vi "Analyzer.DVRtoRef.vi"(10 "Ref":T1) -> (2 "Ref":u32 format="%08x")   [LabVIEW 2022 SP3, in "Analyzer.lvclass"]
uses:
  Analyzer.lvclass
  Typedefs/PrivateData--Ref.ctl
  Typedefs/PrivateData--Cluster.ctl
  Typedefs/PublicEvents--Cluster.ctl
  Typedefs/Analyzer State--enum.ctl
  Typedefs/PublicEvents--Analyzer.NewEventMessage.ctl
  Typedefs/PrivateEvents--Cluster.ctl
  Typedefs/PrivateEvents--Analyzer.NewRequest.ctl
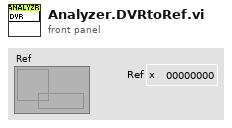
[diagram p1: front panel]
types:
  T1 = typedef "Analyzer.lvclass/PrivateData--Ref.ctl" = refnum<data-value>
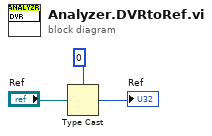
[diagram p0: block diagram]
diagram:
  n1 = Type Cast(type=u32 0 ("Ref"), x="Ref") -> (*(type *) &x=→"Ref":u32)
